vi "Set_ADAM_Watchdog_Timer.vi"() -> ()   [LabVIEW 2010]
panel:
  out "Reply":string
  in  "Watchdog Timer (0000 - 9999)":i32 min=0 max=9999
  in  "Port Name":string="MainNetwork"
  in  "Module Address":i32
  out "String":string
  # "Happy reply starts \"!\"\nUnhappy reply starts \"?\""
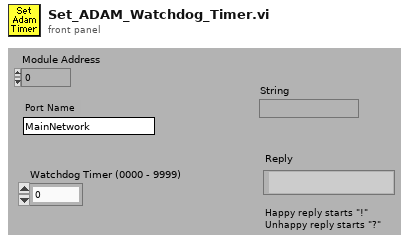
[diagram p1: front panel]
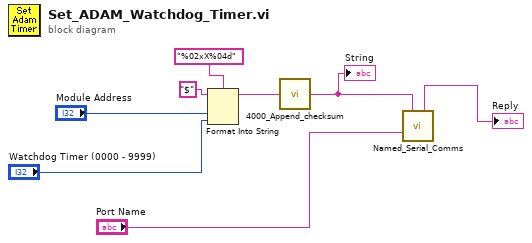
[diagram p0: block diagram]
diagram:
  n1 = Format Into String(format string="%02xX%04d", initial string="$", "Module Address", "Watchdog Timer (0000 - 9999)") -> (resulting string=w4:string)  [unwired: 1 in, 1 out]
  n2 = call "4000_Append_checksum.vi"("ADAM command"=w4) -> ("ADAM string to send"=w1:string)
  "String" <- w1
  n3 = call "Named_Serial_Comms.vi"("Write String"=w1, "Port Name"="Port Name") -> ("Read"=→"Reply":string)  [unwired: 10 in, 3 out]
